vi "FinalProjetVI.vi"() -> ()   [LabVIEW 2018]
uses:
  User32.dll
panel:
  out "Numeric 2":dbl
  out "Numeric":dbl
  out "Filtered Signal 2":dbl
  out "Filtered Signal":dbl
  in  "Accelerometer Sensitivity (mV/g) 2":dbl
  in  "Nominal Zero-g Voltage 2":dbl
  out "data":bool[](array[boolean])
  in  "Accelerometer Sensitivity (mV/g)":dbl
  in  "Nominal Zero-g Voltage":dbl
  out "Waveform Chart":dynamicdata(graph)
  in  "stop (F)":bool
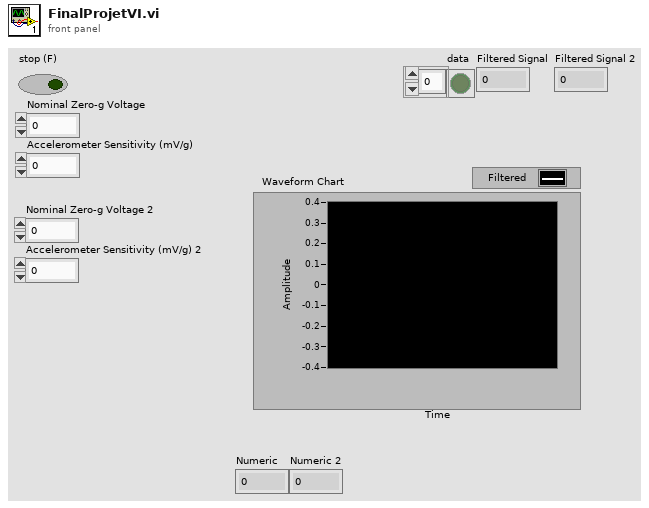
[diagram p1: front panel]
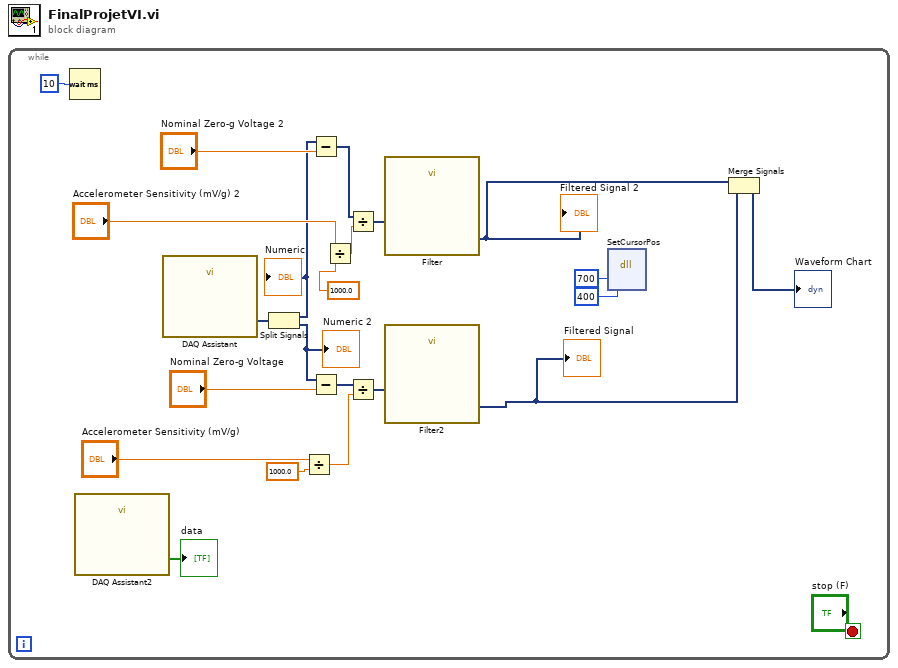
[diagram p0: block diagram]
diagram:
  n1 = while {
    stop <- "stop (F)" stop-if-true
    n2 = Wait (ms)(milliseconds to wait=u32 10) -> ()  [unwired: 1 out]
    n3 = call "DAQ Assistant2"() -> ("data"=→"data":bool[])  [unwired: 17 in, 2 out]
    n4 = call "DAQ Assistant"() -> ("data"=w15:dynamicdata)  [unwired: 17 in, 2 out]
    n5 = Split Signals(w15) -> (w9:dynamicdata, w8:dynamicdata)  [unwired: 2 in]
    "Numeric" <- w9
    "Numeric 2" <- w8
    n6 = Divide(x="Accelerometer Sensitivity (mV/g)", y=1000.0) -> (x/y=w18:dbl)
    n7 = Subtract(x=w9, y="Nominal Zero-g Voltage 2") -> (x-y=w13:dynamicdata)
    n8 = Subtract(x=w8, y="Nominal Zero-g Voltage") -> (x-y=w21:dynamicdata)
    n9 = Divide(x="Accelerometer Sensitivity (mV/g) 2", y=1000.0) -> (x/y=w10:dbl)
    n10 = Divide(x=w13, y=w10) -> (x/y=w6:dynamicdata)
    n11 = Divide(x=w21, y=w18) -> (x/y=w7:dynamicdata)
    n12 = call "Filter"("Signal"=w6) -> ("Filtered Signal"=w5:dynamicdata)  [unwired: 9 in, 1 out]
    "Filtered Signal 2" <- w5
    n13 = call "Filter2"("Signal"=w7) -> ("Filtered Signal"=w3:dynamicdata)  [unwired: 9 in, 1 out]
    "Filtered Signal" <- w3
    n14 = dll-call lib="user32.dll" fn="SetCursorPos"("dx"=700, "dy"=400) -> ()  [unwired: 6 in, 2 out]
    n15 = Merge Signals(w5, w3) -> (→"Waveform Chart":dynamicdata)
  }
